vi "create map.vi"() -> ()   [LabVIEW 2015]
panel:
  out "Map dimensions":dbl[](array[numeric])
  out "Actual robot location":dbl[](array[numeric])
  out "Robot angle":dbl
  out "Obsticle map 2":u16[][](array[ring])
  in  "Obsticle map":u16[][](array[ring])
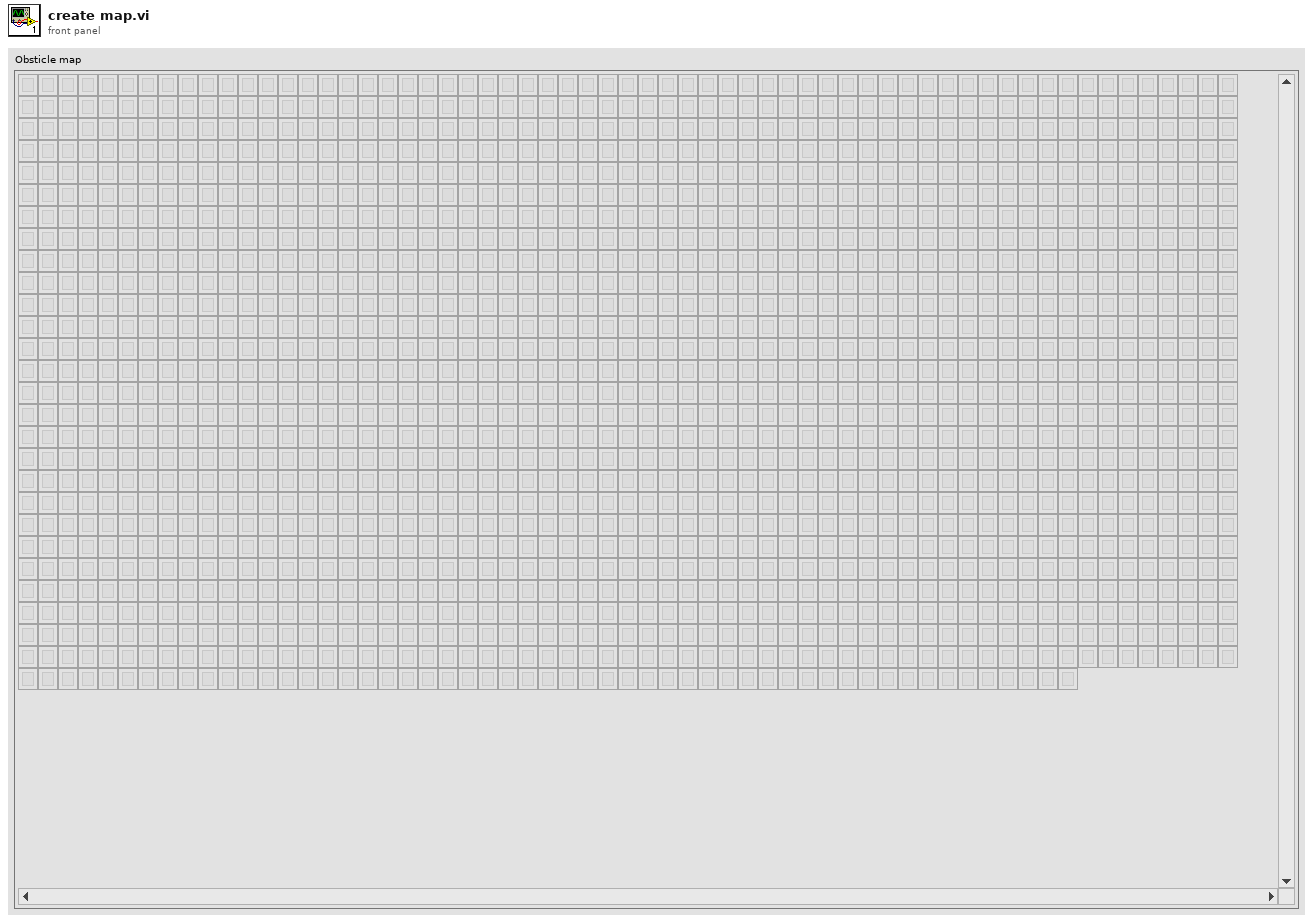
[diagram p1: front panel]
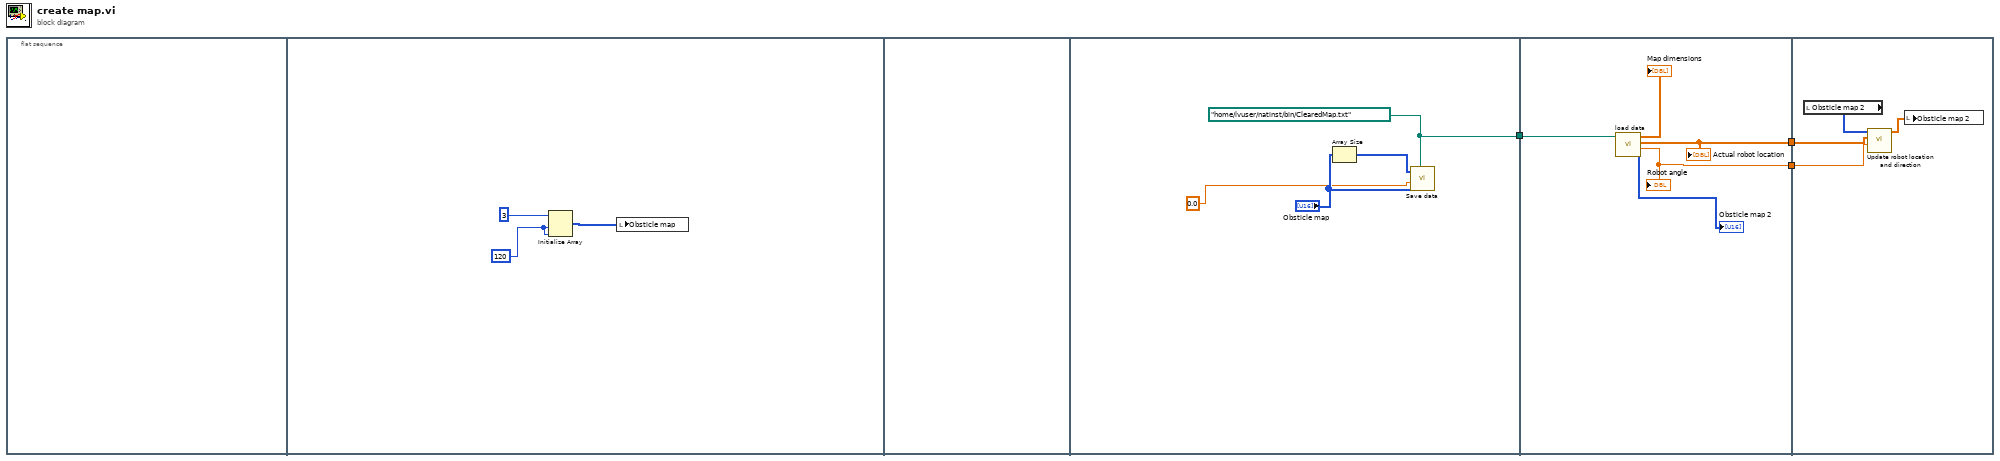
[diagram p0: block diagram]
diagram:
  n1 = flat-sequence {
    tunnel: [w8] -> w1
    tunnel: [w13] -> w3
    tunnel: [w12] -> w2
    tunnel: w1 -> [w11]
    tunnel: w3 -> [w17]
    tunnel: w2 -> [w16]
    frame #0 {
    }
    frame #1 {
      w4 = 120
      n2 = Initialize Array(3, w4, w4) -> (w5:i32[][])
      n3 = local write "Obsticle map"(w5) -> ()
    }
    frame #2 {
    }
    frame #3 {
      w8 = path "/home/lvuser/natinst/bin/ClearedMap.txt" ("file path (use dialog)")
      n4 = Array Size(array="Obsticle map") -> (size(s)=w9:i32[])
      n5 = call "Save data.vi"("file path (use dialog)"=w8, "Obsticle map"="Obsticle map", "Robot angle"=0.0, "Map dimensions"=w9) -> ()  [unwired: 8 in]
    }
    frame #4 {
      n6 = call "load data.vi"("file path (use dialog)"=w11) -> ("Obsticle map"=→"Obsticle map 2":u16[][], "Robot angle"=w12:dbl, "Actual robot location"=w13:dbl[], "Map dimensions"=→"Map dimensions":dbl[])  [unwired: 7 in]
      "Robot angle" <- w12
      "Actual robot location" <- w13
    }
    frame #5 {
      n7 = local read "Obsticle map 2"() -> (w18:u16[][])
      n8 = call "Update robot location and direction.vi"("Map input"=w18, "Actual robot location"=w17, "Robot angle"=w16) -> ("Map Output"=w19:dbl[][])  [unwired: 6 in, 1 out]
      n9 = local write "Obsticle map 2"(w19) -> ()
    }
  }
